vi "Get data folder.vi"() -> (0 "Data folder":path)   [LabVIEW 2015, in "Tests.lvlib"]
uses:
  Tests.lvlib
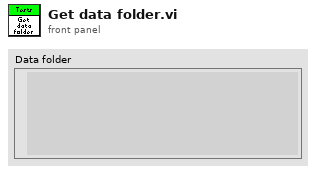
[diagram p1: front panel]
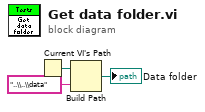
[diagram p0: block diagram]
diagram:
  n1 = Current VI's Path() -> (path=w3:path)
  n2 = Build Path(base path=w3, name or relative path="..\\..\\data") -> (appended path=→"Data folder":path)
